vi "Sort Library Child Data.vi"(8 "Error In":errorcluster, 11 "Unsorted In":refnum<class "Map.lvclass">[](array[class])) -> (0 "Error Out":errorcluster, 3 "Sorted Out":refnum<class "Map.lvclass">[](array[class]))   [LabVIEW 2018, in "Scripts.lvlib"]
uses:
  Scripts.lvlib
  Toolkit/Data/Map/Map.lvclass
  Toolkit/Data/String/String.lvclass
  Toolkit/Data/String/String.lvclass/String.ctl
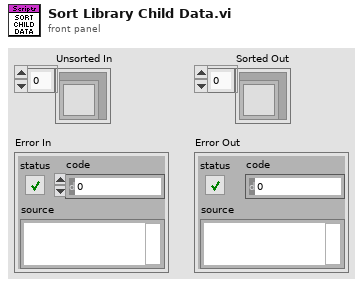
[diagram p1: front panel]
types:
  T1 = cluster{"Value":string, "Map Out":refnum<class "Map.lvclass">}
  T2 = cluster{"Value":string, "Map Out":refnum<class "Map.lvclass">}[]
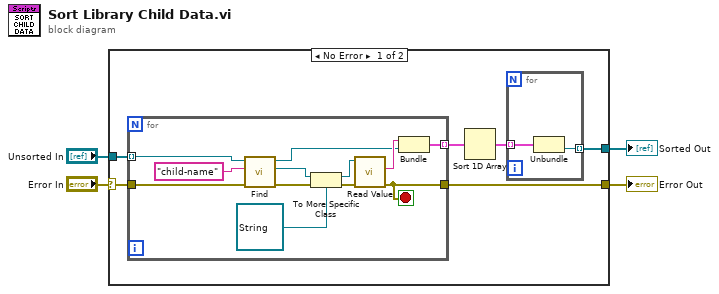
[diagram p0: block diagram]
diagram:
  n1 = case shown="No Error" "Error In" {
    selector: "Error In" -> [w5 w25]
    tunnel: [w10 w26] -> w4
    tunnel: [w8 w25] -> w3
    tunnel: "Unsorted In" -> [w6 w26]
    frame No Error {
      n2 = for {
        tunnel: w6 -> [w24] mode=indexing
        tunnel: w5 -> [w22]
        tunnel: [w14] -> w8
        tunnel: [w13] -> w7 mode=indexing
        stop <- w14 stop-if-true
        n3 = call "Find.vi"("Error In"=w22, "Key"="child-name", "Map In"=w24) -> ("Error Out"=w17:errorcluster, "Value"=w21:refnum<class "Datum.lvclass">, "Map Out"=w15:refnum<class "Map.lvclass">)  [unwired: 5 in, 1 out]
        n4 = To More Specific Class(target class=refnum<class "String.lvclass"> refnum ("Toolkit.lvlib:Data.lvlib:String.lvclass"), reference=w21, error in=w17) -> (specific class reference=w19:refnum<class "String.lvclass">, error out=w18:errorcluster)
        n5 = call "Read Value.vi"("Error In"=w18, "String In"=w19) -> ("Error Out"=w14:errorcluster, "Value"=w16:string)  [unwired: 7 in, 1 out]
        n6 = Bundle("Value"=w16, "Map Out"=w15) -> (w13:T1)  [unwired: 1 in]
      }
      n7 = Sort 1D Array(array=w7) -> (sorted array=w9:T2)
      n8 = for {
        tunnel: w9 -> [w12] mode=indexing
        tunnel: [w11] -> w10 mode=indexing
        n9 = Unbundle(w12) -> ("Map Out"=w11:refnum<class "Map.lvclass">)  [unwired: 1 out]
      }
    }
    frame Error {
    }
  }
  "Sorted Out" <- w4
  "Error Out" <- w3
